vi "CrawlingMotionAlgorithm.vi"() -> ()   [LabVIEW 2018]
doc: "This example demonstrates how to control a servo using LINX."
uses:
  <vilib>/MakerHub/LINX/Public/Utilities/Open Serial.vi
  <vilib>/MakerHub/LINX/Public/Sensors/Motion/Servo/Servo Open One Channel.vi
  <vilib>/MakerHub/LINX/Public/Sensors/Motion/Servo/Servo Set Pulse Width One Channel.vi
  <vilib>/MakerHub/LINX/Public/Sensors/Motion/Servo/Servo Close One Channel.vi
  <vilib>/MakerHub/LINX/LMH-LINX.lvlib
  <vilib>/MakerHub/LINX/Public/Sensors/Motion/Servo/Servo.lvlib
  <vilib>/MakerHub/LINX/Public/Sensors/Distance/Ultrasonic/Ultrasonic.lvlib
panel:
  out "Distanta cm":dbl(slide) scale=0.0..20.0
  in  "Servo Channel 6":u16
  in  "Servo Position 3":u16(knob)=1493 caption="Servo Position" scale=0.0..2.0
  in  "Servo Position 2":u16(knob)=1493 caption="Servo Position" scale=0.0..2.0
  in  "Servo Channel 5":u16
  in  "Servo Channel 7":u16
  in  "Servo Position 1":u16(knob)=1493 caption="Servo Position" scale=0.0..2.0
  out "Loop Rate (Hz)":u32
  in  "Stop Button":bool
  in  "Serial Port":refnum<visa-resource-name>
  # "Neutru/Inainte/Inapoi"
  # "Neutru/Dreapta/Stanga"
  # "Rostogolire\nNeutru/Dreapta/Stanga"
  # "LINX Device Settings"
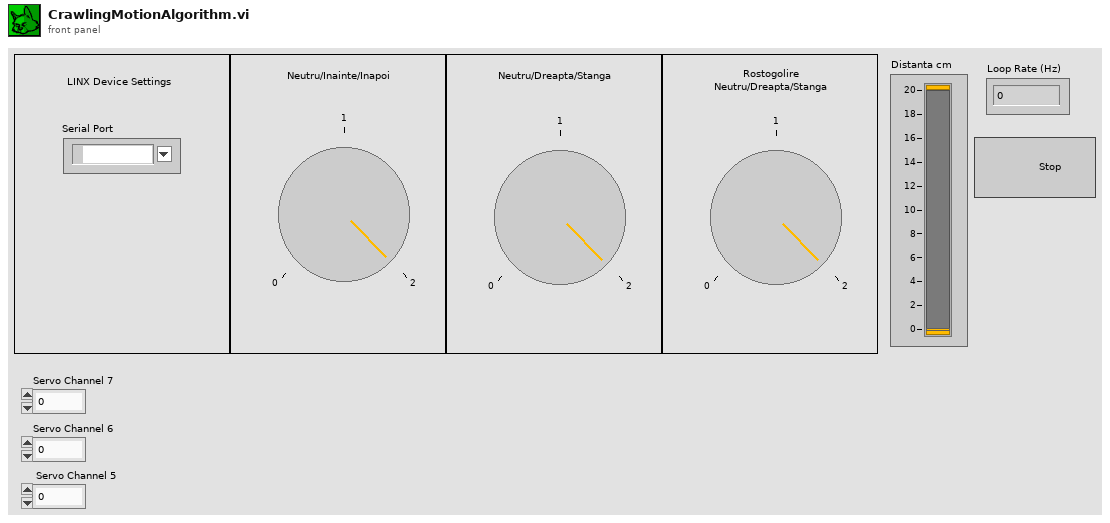
[diagram p1: front panel]
types:
  T1 = typedef "LMH-LINX.lvlib/LINX Ref.ctl" = cluster{"IO":T2, "Interface":T3, "LINX Device Config":T4}
  T2 = typedef "LMH-LINX.lvlib/Platform.ctl" = enum16{"Remote", "Local"}
  T3 = typedef "LMH-LINX.lvlib/Interface.ctl" = enum16{"Serial", "TCP"}
  T4 = typedef "LMH-LINX.lvlib/Device.lvlib/LINX Device Config.ctl" = cluster{"Interface":T3, "COM Port":refnum<visa-resource-name>, "TCP Configuration":T5, "Device Family":u8, "Device ID":u8, "Device Name":string, "TCP Ref":refnum<k5>, "Channels":T6}
  T5 = typedef "LMH-LINX.lvlib/Device.lvlib/TCP Config.ctl" = cluster{"IP Address":string, "Port":u16}
  T6 = typedef "LMH-LINX.lvlib/Channels.ctl" = cluster{"DI":u8[], "DO":u8[], "AI":u8[], "AO":u8[], "PWM":u8[], "QE":u8[], "UART":u8[], "I2C 2":u8[], "SPI":u8[], "CAN":u8[], "Servo":u8[], "AI Ref (V)":dbl, "AI Resolution (Bits)":u8, "AO Ref (V)":dbl, "AO Resolution (Bits)":u8}
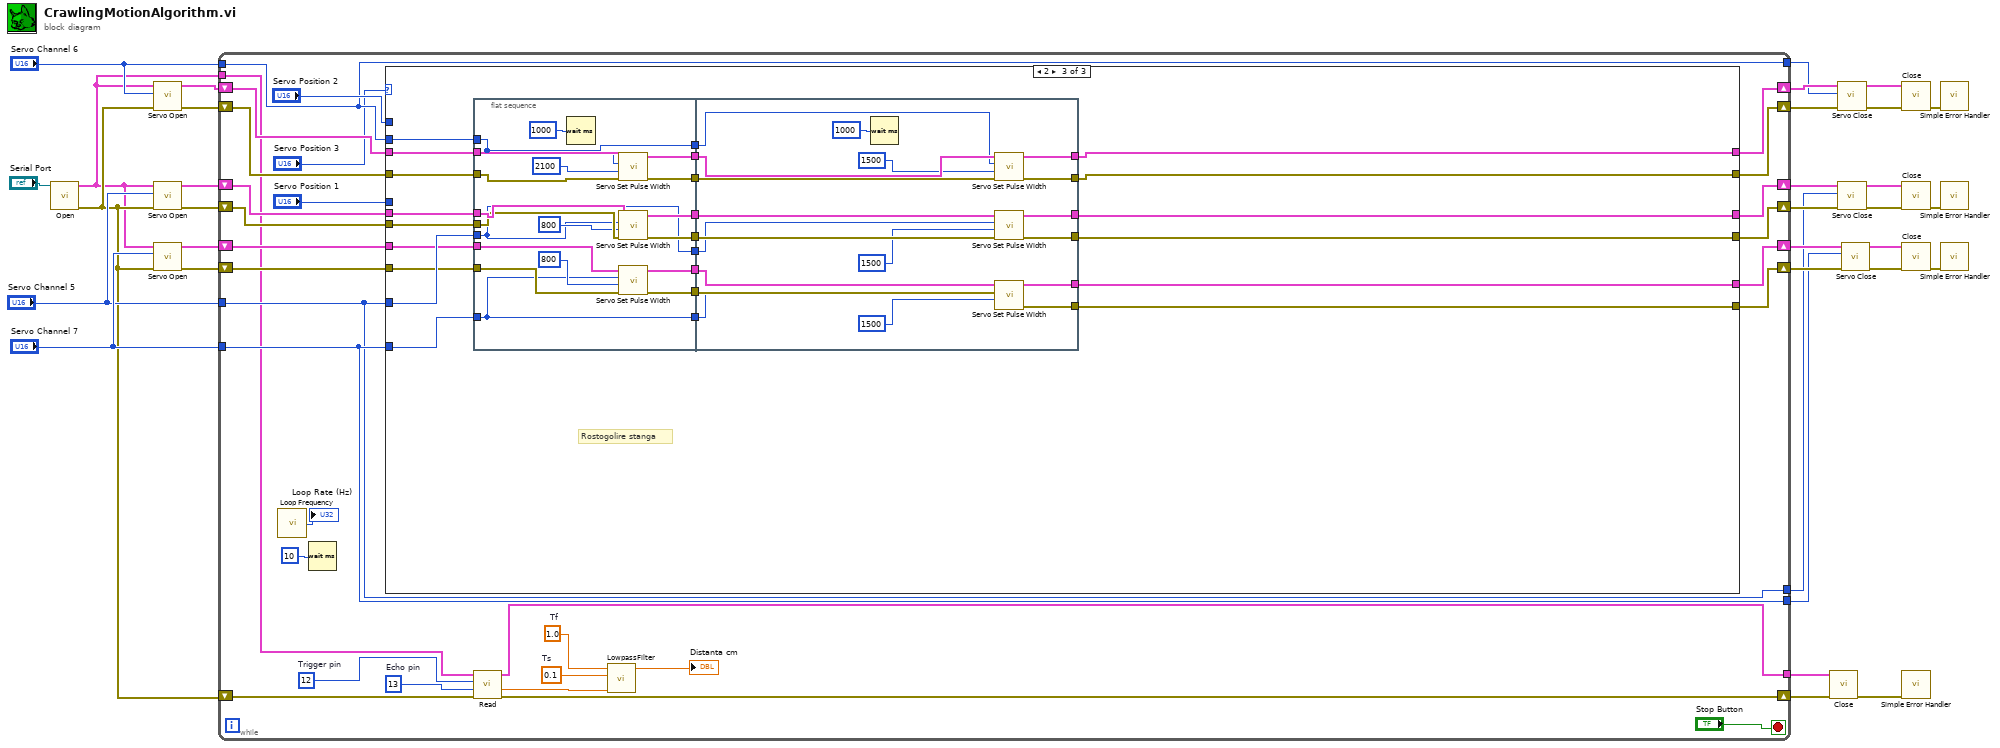
[diagram p0: block diagram]
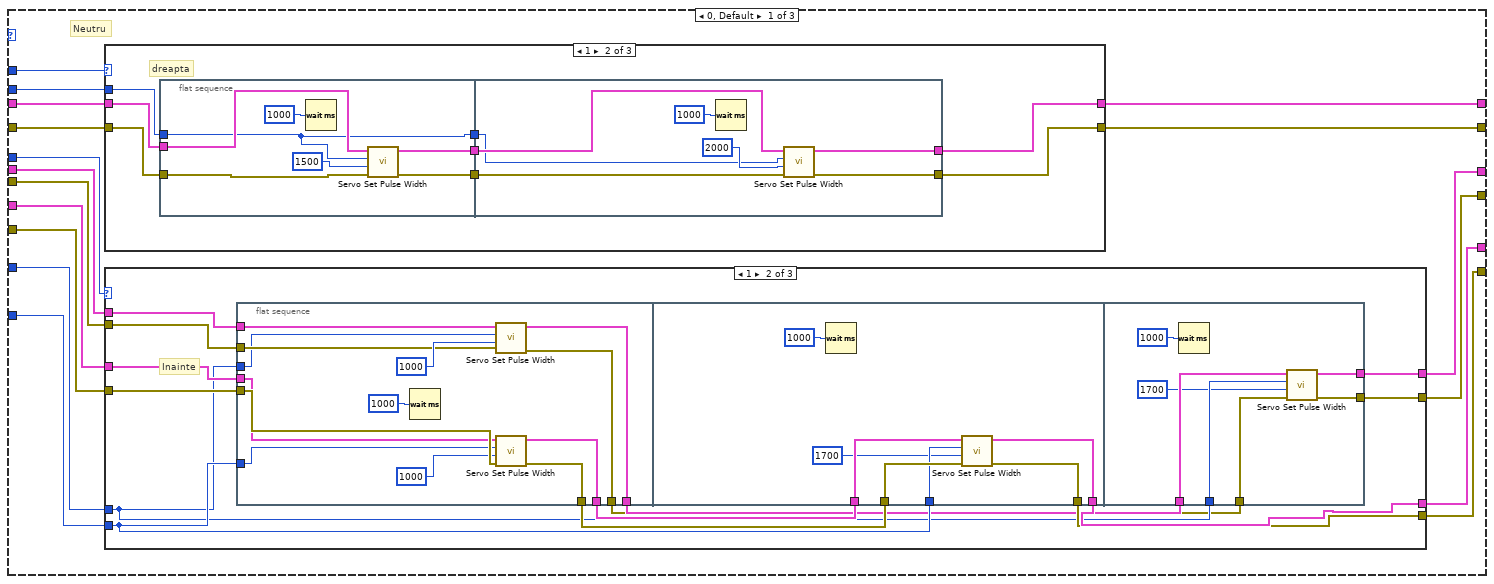
[diagram p2: hidden frame]
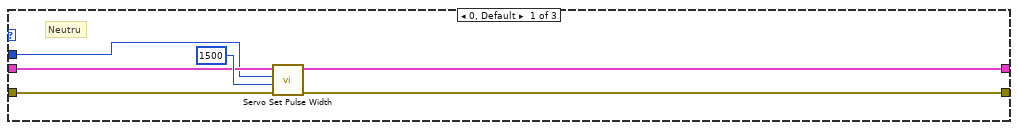
[diagram p3: hidden frame]
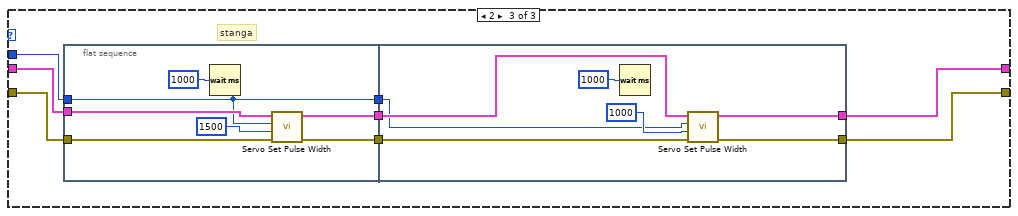
[diagram p4: hidden frame]
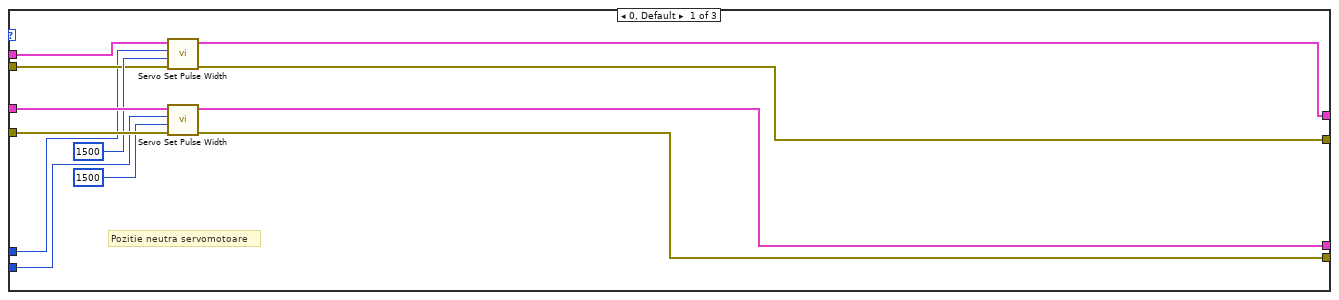
[diagram p5: hidden frame]
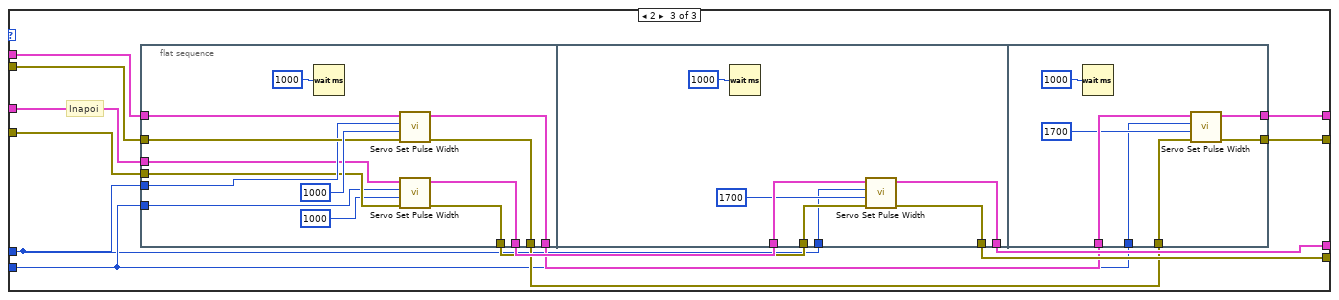
[diagram p6: hidden frame]
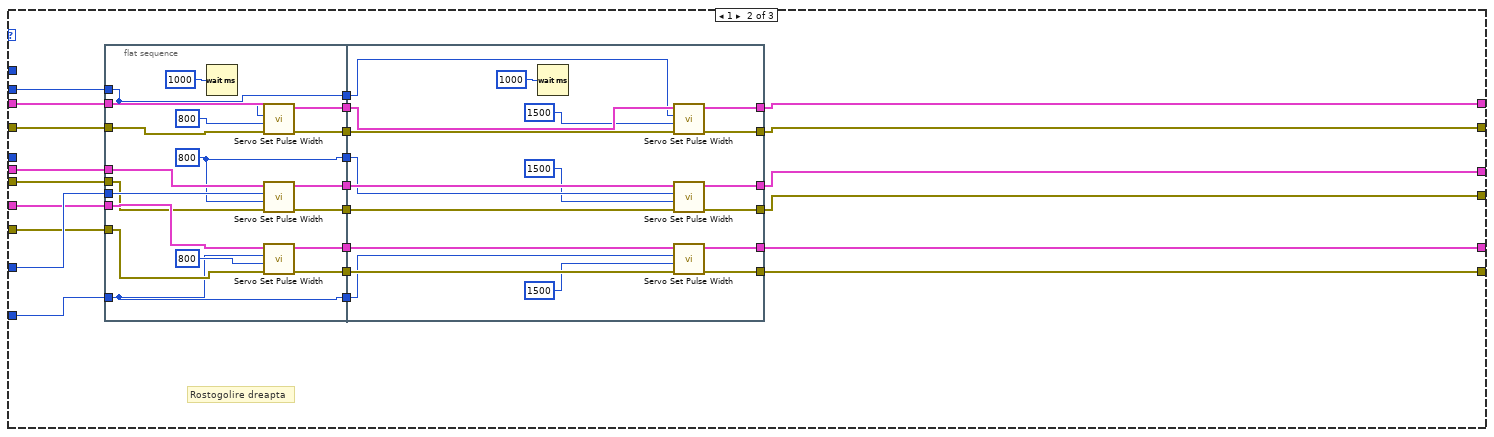
[diagram p7: hidden frame]
diagram:
  n1 = call-poly <vilib>:"Open.vi"("Serial Port"="Serial Port") -> ("Error Out"=w5:errorcluster, "LINX Resource"=w4:T1)  [unwired: 8 in, 1 out]
  n2 = call-poly <vilib>:"Servo Open.vi"("Error In"=w5, "Servo Channel"="Servo Channel 6", "LINX Resource"=w4) -> ("Error Out"=w13:errorcluster, "LINX Resource"=w14:T1)  [unwired: 7 in]
  n3 = call-poly <vilib>:"Servo Open.vi"("Error In"=w5, "Servo Channel"="Servo Channel 5", "LINX Resource"=w4) -> ("Error Out"=w22:errorcluster, "LINX Resource"=w23:T1)  [unwired: 7 in]
  n4 = call-poly <vilib>:"Servo Open.vi"("Error In"=w5, "Servo Channel"="Servo Channel 7", "LINX Resource"=w4) -> ("Error Out"=w32:errorcluster, "LINX Resource"=w31:T1)  [unwired: 7 in]
  n5 = while {
    shift-right: [w56] -> w26
    shift-left: w32 -> [w64]
    tunnel: "Servo Channel 7" -> [w59]
    shift-right: [w62] -> w29
    shift-left: w31 -> [w63]
    tunnel: [w59] -> w25
    shift-right: [w53] -> w18
    shift-left: w23 -> [w57]
    shift-right: [w52] -> w17
    shift-left: w22 -> [w55]
    tunnel: [w54] -> w15
    tunnel: "Servo Channel 5" -> [w54]
    shift-right: [w47] -> w8
    shift-left: w14 -> [w49]
    shift-right: [w46] -> w7
    shift-left: w13 -> [w48]
    tunnel: "Servo Channel 6" -> [w45]
    tunnel: [w45] -> w6
    tunnel: w4 -> [w42]
    tunnel: [w41] -> w2
    shift-right: [w34] -> w1
    shift-left: w5 -> [w43]
    stop <- "Stop Button" stop-if-true
    w40 = 0.1  # Ts
    w39 = 1.0  # Tf
    w35 = u8 13  # Echo pin
    w36 = u8 12  # Trigger pin
    n6 = call <vilib>:"Loop Frequency.vi"() -> ("Loop Rate (Hz)"=→"Loop Rate (Hz)":u32)
    n7 = Wait (ms)(milliseconds to wait=u32 10) -> ()  [unwired: 1 out]
    n8 = case shown="2" "Servo Position 3" {
      tunnel: w64 -> [w81 w241 w303]
      tunnel: w63 -> [w80 w244 w306]
      tunnel: [w79 w229 w292] -> w62
      tunnel: w59 -> [w78 w247 w309]
      tunnel: "Servo Position 1" -> [w65 _ _]
      tunnel: w57 -> [w77 w243 w305]
      tunnel: [w76 w228 w291] -> w56
      tunnel: w55 -> [w75 w242 w304]
      tunnel: w54 -> [w74 w246 w308]
      tunnel: [w73 w231 w294] -> w53
      tunnel: [w72 w230 w293] -> w52
      tunnel: "Servo Position 2" -> [w71 _ _]
      tunnel: w49 -> [w70 w245 w307]
      tunnel: w48 -> [w69 w248 w310]
      tunnel: [w68 w227 w290] -> w47
      tunnel: [w67 w226 w289] -> w46
      tunnel: w45 -> [w66 w249 w311]
      frame 0, Default {
        # "Neutru"
        n9 = case shown="1" w71 {
          tunnel: w70 -> [w83 w95 w112]
          tunnel: w69 -> [w86 w94 w111]
          tunnel: w66 -> [w82 w93 w110]
          tunnel: [w84 w90 w114] -> w68
          tunnel: [w85 w89 w113] -> w67
          frame 0, Default {
            # "Neutru"
            n10 = call-poly <vilib>:"Servo Set Pulse Width.vi"("Error In"=w86, "Pulse Width (uS)"=1500, "Servo Channel"=w82, "LINX Resource"=w83) -> ("Error Out"=w85:errorcluster, "LINX Resource"=w84:T1)  [unwired: 6 in]
          }
          frame 1 {
            # "dreapta"
            n11 = flat-sequence {
              tunnel: w95 -> [w102]
              tunnel: w94 -> [w101]
              tunnel: w93 -> [w97]
              tunnel: [w99] -> w92
              tunnel: [w98] -> w91
              tunnel: [w97] -> w88
              tunnel: w92 -> [w109]
              tunnel: w91 -> [w108]
              tunnel: [w107] -> w90
              tunnel: [w106] -> w89
              tunnel: w88 -> [w104]
              frame #0 {
                n12 = Wait (ms)(milliseconds to wait=u32 1000) -> ()  [unwired: 1 out]
                n13 = call-poly <vilib>:"Servo Set Pulse Width.vi"("Error In"=w101, "Pulse Width (uS)"=1500, "Servo Channel"=w97, "LINX Resource"=w102) -> ("Error Out"=w98:errorcluster, "LINX Resource"=w99:T1)  [unwired: 6 in]
              }
              frame #1 {
                n14 = Wait (ms)(milliseconds to wait=u32 1000) -> ()  [unwired: 1 out]
                n15 = call-poly <vilib>:"Servo Set Pulse Width.vi"("Error In"=w108, "Pulse Width (uS)"=2000, "Servo Channel"=w104, "LINX Resource"=w109) -> ("Error Out"=w106:errorcluster, "LINX Resource"=w107:T1)  [unwired: 6 in]
              }
            }
          }
          frame 2 {
            # "stanga"
            n16 = flat-sequence {
              tunnel: w112 -> [w124]
              tunnel: w111 -> [w123]
              tunnel: w110 -> [w119]
              tunnel: [w121] -> w117
              tunnel: [w120] -> w116
              tunnel: [w119] -> w115
              tunnel: w117 -> [w131]
              tunnel: w116 -> [w130]
              tunnel: [w129] -> w114
              tunnel: [w128] -> w113
              tunnel: w115 -> [w126]
              frame #0 {
                n17 = Wait (ms)(milliseconds to wait=u32 1000) -> ()  [unwired: 1 out]
                n18 = call-poly <vilib>:"Servo Set Pulse Width.vi"("Error In"=w123, "Pulse Width (uS)"=1500, "Servo Channel"=w119, "LINX Resource"=w124) -> ("Error Out"=w120:errorcluster, "LINX Resource"=w121:T1)  [unwired: 6 in]
              }
              frame #1 {
                n19 = Wait (ms)(milliseconds to wait=u32 1000) -> ()  [unwired: 1 out]
                n20 = call-poly <vilib>:"Servo Set Pulse Width.vi"("Error In"=w130, "Pulse Width (uS)"=1000, "Servo Channel"=w126, "LINX Resource"=w131) -> ("Error Out"=w128:errorcluster, "LINX Resource"=w129:T1)  [unwired: 6 in]
              }
            }
          }
        }
        n21 = case shown="1" w65 {
          tunnel: w81 -> [w141 w157 w198]
          tunnel: w80 -> [w143 w156 w197]
          tunnel: [w142 w151 w193] -> w79
          tunnel: w78 -> [w140 w153 w186]
          tunnel: w77 -> [w136 w155 w196]
          tunnel: [w138 w149 w191] -> w76
          tunnel: w75 -> [w135 w154 w195]
          tunnel: w74 -> [w134 w146 w185]
          tunnel: [w133 w147 w189] -> w73
          tunnel: [w132 w145 w188] -> w72
          frame 0, Default {
            # "Pozitie neutra servomotoare"
            n22 = call-poly <vilib>:"Servo Set Pulse Width.vi"("Error In"=w135, "Pulse Width (uS)"=1500, "Servo Channel"=w134, "LINX Resource"=w136) -> ("Error Out"=w132:errorcluster, "LINX Resource"=w133:T1)  [unwired: 6 in]
            n23 = call-poly <vilib>:"Servo Set Pulse Width.vi"("Error In"=w141, "Pulse Width (uS)"=1500, "Servo Channel"=w140, "LINX Resource"=w143) -> ("Error Out"=w138:errorcluster, "LINX Resource"=w142:T1)  [unwired: 6 in]
          }
          frame 1 {
            # "Inainte"
            n24 = flat-sequence {
              tunnel: w155 -> [w168]
              tunnel: w154 -> [w167]
              tunnel: [w166] -> w144
              tunnel: [w165] -> w148
              tunnel: w146 -> [w164]
              tunnel: [w158] -> w150
              tunnel: [w159] -> w152
              tunnel: w153 -> [w161]
              tunnel: w156 -> [w162]
              tunnel: w157 -> [w163]
              tunnel: w152 -> [w177]
              tunnel: w150 -> [w176]
              tunnel: w153 -> [w175]
              tunnel: [w172] -> w151
              tunnel: [w171] -> w149
              tunnel: w148 -> [w184]
              tunnel: [w183] -> w147
              tunnel: w146 -> [w182]
              tunnel: w144 -> [w179]
              tunnel: [w178] -> w145
              frame #0 {
                n25 = Wait (ms)(milliseconds to wait=u32 1000) -> ()  [unwired: 1 out]
                n26 = call-poly <vilib>:"Servo Set Pulse Width.vi"("Error In"=w167, "Pulse Width (uS)"=1000, "Servo Channel"=w164, "LINX Resource"=w168) -> ("Error Out"=w166:errorcluster, "LINX Resource"=w165:T1)  [unwired: 6 in]
                n27 = call-poly <vilib>:"Servo Set Pulse Width.vi"("Error In"=w163, "Pulse Width (uS)"=1000, "Servo Channel"=w161, "LINX Resource"=w162) -> ("Error Out"=w158:errorcluster, "LINX Resource"=w159:T1)  [unwired: 6 in]
              }
              frame #1 {
                n28 = Wait (ms)(milliseconds to wait=u32 1000) -> ()  [unwired: 1 out]
                n29 = call-poly <vilib>:"Servo Set Pulse Width.vi"("Error In"=w176, "Pulse Width (uS)"=1700, "Servo Channel"=w175, "LINX Resource"=w177) -> ("Error Out"=w171:errorcluster, "LINX Resource"=w172:T1)  [unwired: 6 in]
              }
              frame #2 {
                n30 = Wait (ms)(milliseconds to wait=u32 1000) -> ()  [unwired: 1 out]
                n31 = call-poly <vilib>:"Servo Set Pulse Width.vi"("Error In"=w179, "Pulse Width (uS)"=1700, "Servo Channel"=w182, "LINX Resource"=w184) -> ("Error Out"=w178:errorcluster, "LINX Resource"=w183:T1)  [unwired: 6 in]
              }
            }
          }
          frame 2 {
            # "Inapoi"
            n32 = flat-sequence {
              tunnel: w196 -> [w209]
              tunnel: w195 -> [w208]
              tunnel: [w207] -> w187
              tunnel: [w206] -> w190
              tunnel: w185 -> [w205]
              tunnel: [w199] -> w192
              tunnel: [w200] -> w194
              tunnel: w186 -> [w202]
              tunnel: w197 -> [w203]
              tunnel: w198 -> [w204]
              tunnel: w194 -> [w218]
              tunnel: w192 -> [w217]
              tunnel: [w214] -> w193
              tunnel: [w213] -> w191
              tunnel: w185 -> [w212]
              tunnel: w190 -> [w225]
              tunnel: [w224] -> w189
              tunnel: w187 -> [w221]
              tunnel: [w220] -> w188
              tunnel: w186 -> [w219]
              frame #0 {
                n33 = Wait (ms)(milliseconds to wait=u32 1000) -> ()  [unwired: 1 out]
                n34 = call-poly <vilib>:"Servo Set Pulse Width.vi"("Error In"=w208, "Pulse Width (uS)"=1000, "Servo Channel"=w205, "LINX Resource"=w209) -> ("Error Out"=w207:errorcluster, "LINX Resource"=w206:T1)  [unwired: 6 in]
                n35 = call-poly <vilib>:"Servo Set Pulse Width.vi"("Error In"=w204, "Pulse Width (uS)"=1000, "Servo Channel"=w202, "LINX Resource"=w203) -> ("Error Out"=w199:errorcluster, "LINX Resource"=w200:T1)  [unwired: 6 in]
              }
              frame #1 {
                n36 = Wait (ms)(milliseconds to wait=u32 1000) -> ()  [unwired: 1 out]
                n37 = call-poly <vilib>:"Servo Set Pulse Width.vi"("Error In"=w217, "Pulse Width (uS)"=1700, "Servo Channel"=w212, "LINX Resource"=w218) -> ("Error Out"=w213:errorcluster, "LINX Resource"=w214:T1)  [unwired: 6 in]
              }
              frame #2 {
                n38 = Wait (ms)(milliseconds to wait=u32 1000) -> ()  [unwired: 1 out]
                n39 = call-poly <vilib>:"Servo Set Pulse Width.vi"("Error In"=w221, "Pulse Width (uS)"=1700, "Servo Channel"=w219, "LINX Resource"=w225) -> ("Error Out"=w220:errorcluster, "LINX Resource"=w224:T1)  [unwired: 6 in]
              }
            }
          }
        }
      }
      frame 1 {
        # "Rostogolire dreapta"
        n40 = flat-sequence {
          tunnel: w249 -> [w250]
          tunnel: w248 -> [w266]
          tunnel: w247 -> [w253]
          tunnel: w246 -> [w263]
          tunnel: w245 -> [w268]
          tunnel: w244 -> [w265]
          tunnel: w243 -> [w264]
          tunnel: w242 -> [w262]
          tunnel: w241 -> [w261]
          tunnel: [w259] -> w240
          tunnel: [w258] -> w239
          tunnel: [w257] -> w238
          tunnel: [w256] -> w237
          tunnel: [w255] -> w236
          tunnel: [w254] -> w235
          tunnel: [w250] -> w234
          tunnel: [w253] -> w233
          tunnel: [w252] -> w232
          tunnel: w240 -> [w287]
          tunnel: w239 -> [w286]
          tunnel: w238 -> [w285]
          tunnel: w237 -> [w284]
          tunnel: w236 -> [w283]
          tunnel: w235 -> [w282]
          tunnel: w234 -> [w281]
          tunnel: w233 -> [w280]
          tunnel: w232 -> [w279]
          tunnel: [w274] -> w231
          tunnel: [w273] -> w230
          tunnel: [w272] -> w229
          tunnel: [w271] -> w228
          tunnel: [w270] -> w227
          tunnel: [w269] -> w226
          frame #0 {
            w252 = u16 800 ("Pulse Width (uS)")
            n41 = Wait (ms)(milliseconds to wait=u32 1000) -> ()  [unwired: 1 out]
            n42 = call-poly <vilib>:"Servo Set Pulse Width.vi"("Error In"=w266, "Pulse Width (uS)"=u16 800, "Servo Channel"=w250, "LINX Resource"=w268) -> ("Error Out"=w254:errorcluster, "LINX Resource"=w255:T1)  [unwired: 6 in]
            n43 = call-poly <vilib>:"Servo Set Pulse Width.vi"("Error In"=w262, "Pulse Width (uS)"=w252, "Servo Channel"=w263, "LINX Resource"=w264) -> ("Error Out"=w258:errorcluster, "LINX Resource"=w259:T1)  [unwired: 6 in]
            n44 = call-poly <vilib>:"Servo Set Pulse Width.vi"("Error In"=w261, "Pulse Width (uS)"=u16 800, "Servo Channel"=w253, "LINX Resource"=w265) -> ("Error Out"=w257:errorcluster, "LINX Resource"=w256:T1)  [unwired: 6 in]
          }
          frame #1 {
            n45 = Wait (ms)(milliseconds to wait=u32 1000) -> ()  [unwired: 1 out]
            n46 = call-poly <vilib>:"Servo Set Pulse Width.vi"("Error In"=w282, "Pulse Width (uS)"=u16 1500, "Servo Channel"=w281, "LINX Resource"=w283) -> ("Error Out"=w269:errorcluster, "LINX Resource"=w270:T1)  [unwired: 6 in]
            n47 = call-poly <vilib>:"Servo Set Pulse Width.vi"("Error In"=w286, "Pulse Width (uS)"=u16 1500, "Servo Channel"=w279, "LINX Resource"=w287) -> ("Error Out"=w273:errorcluster, "LINX Resource"=w274:T1)  [unwired: 6 in]
            n48 = call-poly <vilib>:"Servo Set Pulse Width.vi"("Error In"=w285, "Pulse Width (uS)"=u16 1500, "Servo Channel"=w280, "LINX Resource"=w284) -> ("Error Out"=w271:errorcluster, "LINX Resource"=w272:T1)  [unwired: 6 in]
          }
        }
      }
      frame 2 {
        # "Rostogolire stanga"
        n49 = flat-sequence {
          tunnel: w311 -> [w316]
          tunnel: w310 -> [w328]
          tunnel: w309 -> [w315]
          tunnel: w308 -> [w312]
          tunnel: w307 -> [w330]
          tunnel: w306 -> [w327]
          tunnel: w305 -> [w326]
          tunnel: w304 -> [w325]
          tunnel: w303 -> [w324]
          tunnel: [w322] -> w302
          tunnel: [w321] -> w301
          tunnel: [w320] -> w300
          tunnel: [w319] -> w299
          tunnel: [w318] -> w298
          tunnel: [w317] -> w297
          tunnel: [w316] -> w296
          tunnel: [w315] -> w295
          tunnel: [w312] -> w288
          tunnel: w302 -> [w349]
          tunnel: w301 -> [w348]
          tunnel: w300 -> [w347]
          tunnel: w299 -> [w346]
          tunnel: w298 -> [w345]
          tunnel: w297 -> [w344]
          tunnel: w296 -> [w343]
          tunnel: w295 -> [w342]
          tunnel: [w336] -> w294
          tunnel: [w335] -> w293
          tunnel: [w334] -> w292
          tunnel: [w333] -> w291
          tunnel: [w332] -> w290
          tunnel: [w331] -> w289
          tunnel: w288 -> [w341]
          frame #0 {
            n50 = Wait (ms)(milliseconds to wait=u32 1000) -> ()  [unwired: 1 out]
            n51 = call-poly <vilib>:"Servo Set Pulse Width.vi"("Error In"=w328, "Pulse Width (uS)"=u16 2100, "Servo Channel"=w316, "LINX Resource"=w330) -> ("Error Out"=w317:errorcluster, "LINX Resource"=w318:T1)  [unwired: 6 in]
            n52 = call-poly <vilib>:"Servo Set Pulse Width.vi"("Error In"=w325, "Pulse Width (uS)"=u16 800, "Servo Channel"=w312, "LINX Resource"=w326) -> ("Error Out"=w321:errorcluster, "LINX Resource"=w322:T1)  [unwired: 6 in]
            n53 = call-poly <vilib>:"Servo Set Pulse Width.vi"("Error In"=w324, "Pulse Width (uS)"=u16 800, "Servo Channel"=w315, "LINX Resource"=w327) -> ("Error Out"=w320:errorcluster, "LINX Resource"=w319:T1)  [unwired: 6 in]
          }
          frame #1 {
            n54 = Wait (ms)(milliseconds to wait=u32 1000) -> ()  [unwired: 1 out]
            n55 = call-poly <vilib>:"Servo Set Pulse Width.vi"("Error In"=w344, "Pulse Width (uS)"=u16 1500, "Servo Channel"=w343, "LINX Resource"=w345) -> ("Error Out"=w331:errorcluster, "LINX Resource"=w332:T1)  [unwired: 6 in]
            n56 = call-poly <vilib>:"Servo Set Pulse Width.vi"("Error In"=w348, "Pulse Width (uS)"=u16 1500, "Servo Channel"=w341, "LINX Resource"=w349) -> ("Error Out"=w335:errorcluster, "LINX Resource"=w336:T1)  [unwired: 6 in]
            n57 = call-poly <vilib>:"Servo Set Pulse Width.vi"("Error In"=w347, "Pulse Width (uS)"=u16 1500, "Servo Channel"=w342, "LINX Resource"=w346) -> ("Error Out"=w333:errorcluster, "LINX Resource"=w334:T1)  [unwired: 6 in]
          }
        }
      }
    }
    n58 = call <vilib>:"Read.vi"("Error In"=w43, "DO Channel"=w35, "DI Channel"=w36, "LINX Resource"=w42) -> ("Error Out"=w34:errorcluster, "Centimeters"=w37:dbl, "LINX Resource"=w41:T1)  [unwired: 4 in, 1 out]
    n59 = call "LowpassFilter.vi"("ln_k"=w37, "Ts"=w40, "Tf"=w39) -> ("Filter output"=→"Distanta cm":dbl)  [unwired: 8 in]
  }
  n60 = call <vilib>:"Close.vi"("Error In"=w1, "LINX Resource"=w2) -> ("Error Out"=w3:errorcluster)  [unwired: 9 in]
  n61 = call-poly <vilib>:"Servo Close.vi"("Error In"=w7, "Servo Channel"=w6, "LINX Resource"=w8) -> ("Error Out"=w9:errorcluster, "LINX Resource"=w10:T1)  [unwired: 7 in]
  n62 = call-poly <vilib>:"Servo Close.vi"("Error In"=w17, "Servo Channel"=w15, "LINX Resource"=w18) -> ("Error Out"=w19:errorcluster, "LINX Resource"=w20:T1)  [unwired: 7 in]
  n63 = call-poly <vilib>:"Servo Close.vi"("Error In"=w26, "Servo Channel"=w25, "LINX Resource"=w29) -> ("Error Out"=w27:errorcluster, "LINX Resource"=w28:T1)  [unwired: 7 in]
  n64 = call <vilib>:"Close.vi"("Error In"=w9, "LINX Resource"=w10) -> ("Error Out"=w11:errorcluster)  [unwired: 9 in]
  n65 = call <vilib>:"Close.vi"("Error In"=w19, "LINX Resource"=w20) -> ("Error Out"=w21:errorcluster)  [unwired: 9 in]
  n66 = call <vilib>:"Close.vi"("Error In"=w27, "LINX Resource"=w28) -> ("Error Out"=w30:errorcluster)  [unwired: 9 in]
  n67 = call <vilib>:"Simple Error Handler.vi"("error in (no error)"=w3) -> ()  [unwired: 4 in, 5 out]
  n68 = call <vilib>:"Simple Error Handler.vi"("error in (no error)"=w11) -> ()  [unwired: 4 in, 5 out]
  n69 = call <vilib>:"Simple Error Handler.vi"("error in (no error)"=w21) -> ()  [unwired: 4 in, 5 out]
  n70 = call <vilib>:"Simple Error Handler.vi"("error in (no error)"=w30) -> ()  [unwired: 4 in, 5 out]
